vi "SICK.vi"() -> ()   [LabVIEW 2015]
uses:
  <instrlib>/Sick LMS 2XX Series/HAIOL/Sick LMS 2XX Series.lvclass
  <instrlib>/Sick LMS 2XX Series/HAIOL/VISA/Sick LMS 2XX Series VISA.lvclass
  <vilib>/robotics/Navigation/shared/WorldMap/OccupancyGridWorldMap/NI_Robotics_OccupancyGridWorldMap.lvclass
panel:
  out "Intensity Graph":dbl[][](graph)
  in  "index":i32=180
  out "element 2":u16
  out "element":dbl
  in  "Baud Rate":u16(ring) items=["9600", "19200", "38400", "500000"]
  in  "VISA resource name":refnum<visa-resource-name>
  out "Reflectivity Values":i32[](array[numeric])
  out "Polar Co-ordinates":u16[](array[numeric])
  in  "LMS Type (0: Standard)":u16(ring) items=["Standard", "Non-Standard"]
  in  "Stop":bool
  in  "Reset":bool
  out "Cartesian Graph":cluster{"X":dbl[], "Y":dbl[]}(graph)
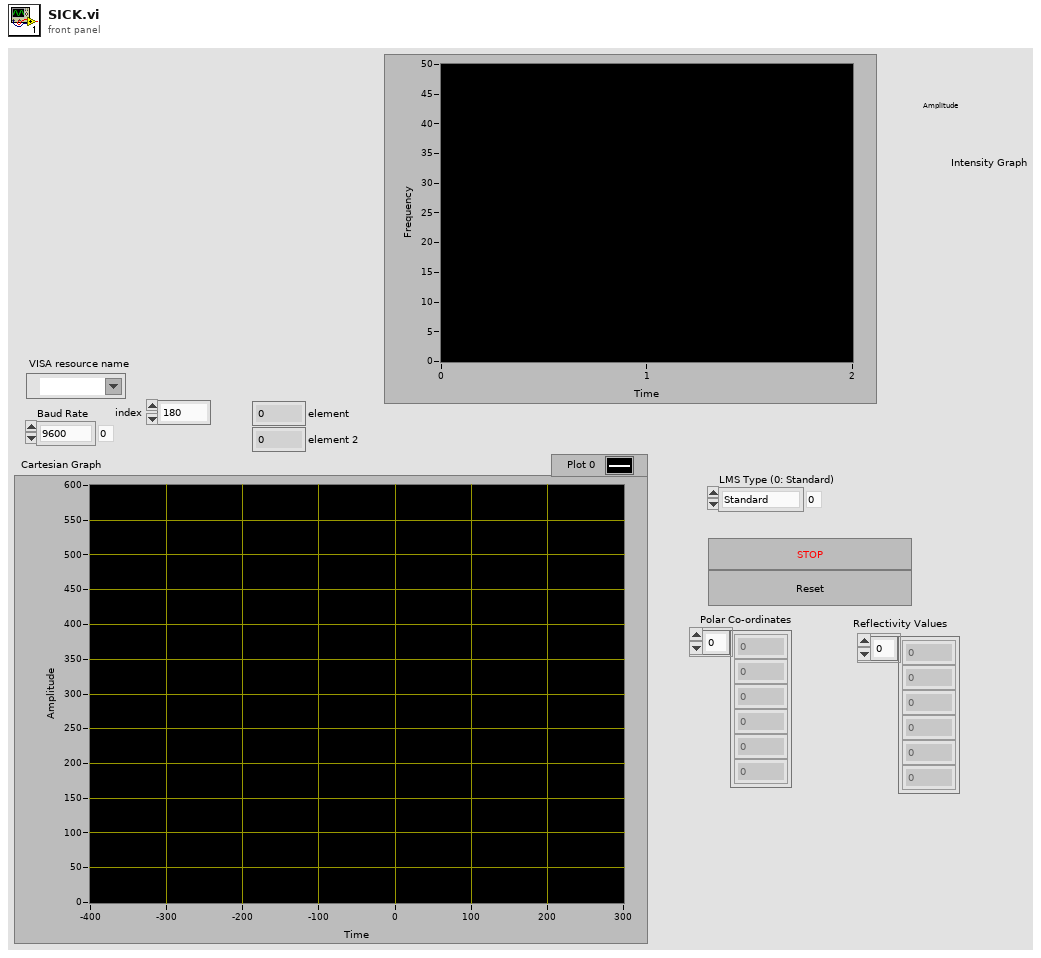
[diagram p1: front panel]
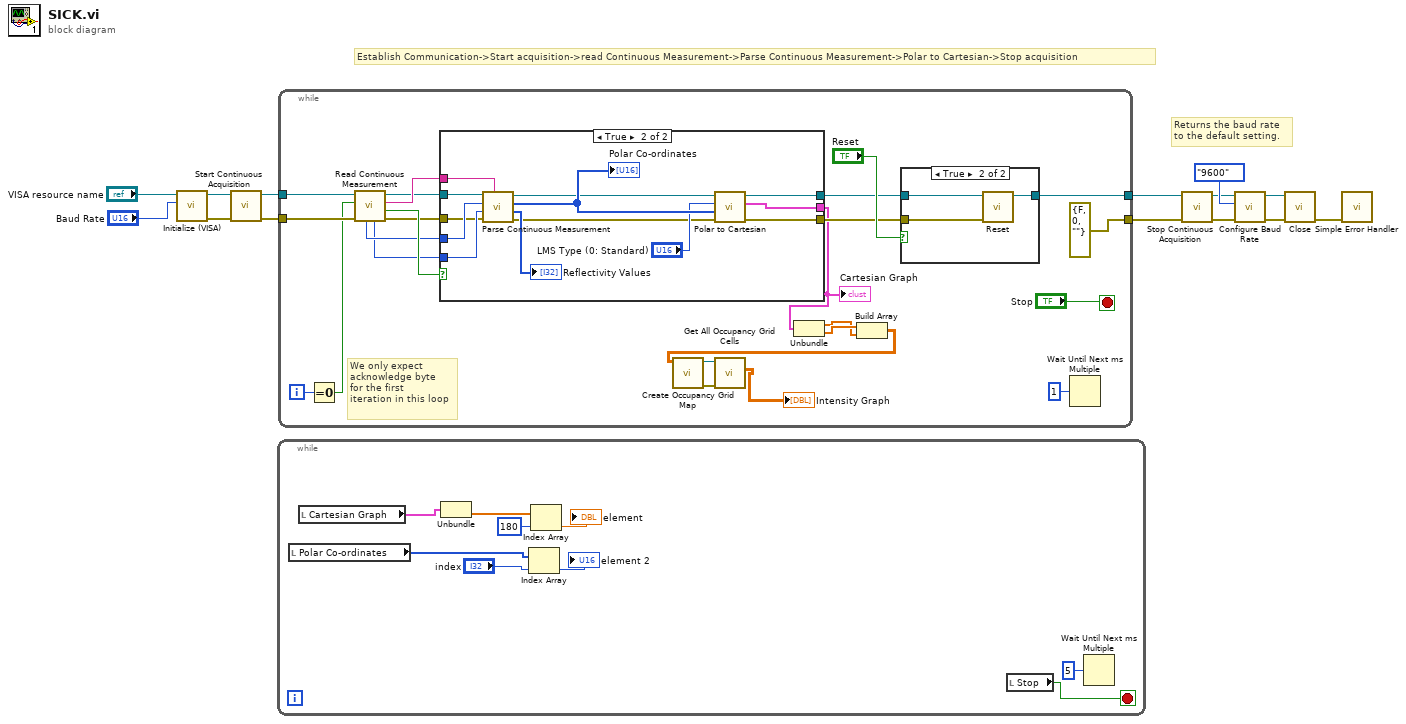
[diagram p0: block diagram]
diagram:
  # "Returns the baud rate to the default setting."
  # "Establish Communication->Start acquisition->read Continuous Measurement->Parse Continuous Measurement->Polar to Cartesian->Stop acquisition"
  n1 = call <instrlib>:"Initialize (VISA).vi"("Baud Rate"="Baud Rate", "VISA resource name"="VISA resource name") -> ("error out"=w4:errorcluster, "Sick LMS 2XX Series out"=w5:refnum<class "Sick LMS 2XX Series.lvclass">)  [unwired: 8 in]
  n2 = call-dynamic "Start Continuous Acquisition.vi"("error in (no error)"=w4, "Sick LMS 2XX Series"=w5) -> ("error out"=w7:errorcluster, "Sick LMS 2XX Series out"=w8:refnum<class "Sick LMS 2XX Series.lvclass">)  [unwired: 8 in]
  n3 = while {
    stop <- w18 stop-if-true
    n4 = local read "Polar Co-ordinates"() -> (w16:u16[])
    n5 = local read "Cartesian Graph"() -> (w23:cluster{"X":dbl[], "Y":dbl[]})
    n6 = Unbundle(w23) -> ("Y"=w22:dbl[])  [unwired: 1 out]
    n7 = Index Array(array=w16, index="index") -> (element=→"element 2":u16)
    n8 = Index Array(array=w22, index=180) -> (element=→"element":dbl)
    n9 = local read "Stop"() -> (w18:bool)
    n10 = Wait Until Next ms Multiple(millisecond multiple=u32 5) -> ()  [unwired: 1 out]
  }
  n11 = while {
    tunnel: [w40] -> w1
    tunnel: [errorcluster {"status"=FALSE, "code"=0, "source"=""} ("error out")] -> w9
    tunnel: w8 -> [w47]
    tunnel: w7 -> [w46]
    i -> [w42]
    stop <- "Stop" stop-if-true
    # "We only expect\nacknowledge byte\nfor the first\niteration in this loop"
    n12 = Equal To 0?(x=w42) -> (x = 0?=w41:bool)
    n13 = call-dynamic "Read Continuous Measurement.vi"("error in (no error)"=w46, "Enable Acknowledge Byte (T: Enable)"=w41, "Sick LMS 2XX Series"=w47) -> ("error out"=w33:errorcluster, "CRC Check"=w44:bool, "Read Buffer"=w45:string, "Sick LMS 2XX Series out"=w34:refnum<class "Sick LMS 2XX Series.lvclass">, "Number of Reflectances"=w38:u16, "Number of Distances"=w39:u16)  [unwired: 2 in, 1 out]
    n14 = case shown="True" w44 {
      tunnel: w45 -> [_ w66]
      tunnel: w39 -> [_ w65]
      tunnel: w38 -> [_ w64]
      tunnel: [_ w62] -> w30
      tunnel: w34 -> [w53 w59]
      tunnel: w33 -> [w52 w58]
      tunnel: [w53 w55] -> w32
      tunnel: [w52 w54] -> w31
      frame False {
        # "If CRC fails, ignore data"
      }
      frame True {
        n15 = call-dynamic "Parse Continuous Measurement.vi"("Input Data"=w66, "error in (no error)"=w58, "Number of Reflectances (0)"=w64, "Number of Measurements (1)"=w65, "Sick LMS 2XX Series"=w59) -> ("error out"=w57:errorcluster, "Reflectivity Values"=→"Reflectivity Values":i32[], "Polar Co-ordinates"=w61:u16[], "Sick LMS 2XX Series out"=w56:refnum<class "Sick LMS 2XX Series.lvclass">)  [unwired: 3 in]
        "Polar Co-ordinates" <- w61
        n16 = call-dynamic "Polar to Cartesian.vi"("error in (no error)"=w57, "Distances"=w61, "LMS Type (0: Standard)"="LMS Type (0: Standard)", "Sick LMS 2XX Series"=w56) -> ("error out"=w54:errorcluster, "Cartesian"=w62:cluster{"X (cm)":dbl[], "Y (cm)":dbl[]}, "Sick LMS 2XX Series out"=w55:refnum<class "Sick LMS 2XX Series.lvclass">)  [unwired: 5 in]
      }
    }
    "Cartesian Graph" <- w30
    n17 = Unbundle(w30) -> ("X (cm)"=w24:dbl[], "Y (cm)"=w25:dbl[])
    n18 = Build Array(w25, w24) -> (w29:dbl[][])
    n19 = call <vilib>:"Create Occupancy Grid Map.vi"("occupancy grid"=w29) -> ("error out"=w27:errorcluster, "map reference out"=w28:refnum<data-value>)  [unwired: 9 in]
    n20 = call <vilib>:"Get All Occupancy Grid Cells.vi"("error in (no error)"=w27, "map reference in"=w28) -> ("occupancy grid"=→"Intensity Graph":dbl[][])  [unwired: 7 in, 2 out]
    n21 = case shown="True" "Reset" {
      tunnel: [w48 w50] -> w40
      tunnel: w32 -> [w48 w51]
      tunnel: w31 -> [_ w49]
      frame False {
      }
      frame True {
        n22 = call-dynamic "Reset.vi"("error in (no error)"=w49, "Sick LMS 2XX Series"=w51) -> ("Sick LMS 2XX Series out"=w50:refnum<class "Sick LMS 2XX Series.lvclass">)  [unwired: 8 in, 1 out]
      }
    }
    n23 = Wait Until Next ms Multiple(millisecond multiple=u32 1) -> ()  [unwired: 1 out]
  }
  n24 = call-dynamic "Stop Continuous Acquisition.vi"("error in (no error)"=w9, "Sick LMS 2XX Series"=w1) -> ("error out"=w12:errorcluster, "Sick LMS 2XX Series out"=w13:refnum<class "Sick LMS 2XX Series.lvclass">)  [unwired: 7 in, 1 out]
  n25 = call-dynamic "Configure Baud Rate.vi"("error in (no error)"=w12, "Baud Rate"=enum16{"9600", "19200", "38400", "500000"}."9600" ("Enum"), "Sick LMS 2XX Series"=w13) -> ("error out"=w10:errorcluster, "Sick LMS 2XX Series out"=w11:refnum<class "Sick LMS 2XX Series.lvclass">)  [unwired: 7 in]
  n26 = call-dynamic "Close.vi"("error in (no error)"=w10, "Sick LMS 2XX Series"=w11) -> ("error out"=w6:errorcluster)  [unwired: 9 in]
  n27 = call <vilib>:"Simple Error Handler.vi"("error in (no error)"=w6) -> ()  [unwired: 4 in, 5 out]
